vi "Read FD.vi"(8 "error in":errorcluster, 11 "TPCANHandle in":T2=81 items=["PCAN_NONEBUS"=0, "PCAN_USBBUS1"=81, "PCAN_USBBUS2"=82, "PCAN_USBBUS3"=83, "PCAN_USBBUS4"=84, "PCAN_USBBUS5"=85, "PCAN_USBBUS6"=86, "PCAN_USBBUS7"=87, "PCAN_USBBUS8"=88, "PCAN_USBBUS9"=1289, "PCAN_USBBUS10"=1290, "PCAN_USBBUS11"=1291, "PCAN_USBBUS12"=1292, "PCAN_USBBUS13"=1293, "PCAN_USBBUS14"=1294, "PCAN_USBBUS15"=1295, "PCAN_USBBUS16"=1296]) -> (0 "error out":errorcluster, 1 "Time Stamp":timestamp format="%<%x %.3X>T", 2 "PCAN Message FD":T3={"ID"=0, "MSGTYPE"={"Type"=4, "Extended"=FALSE, "ESI"=FALSE, "Echo"=FALSE}, "LEN"=enum."0", "Data"=[]} {"Data" format="%.0x"; "MSGTYPE"."Type" items=["FD"=4, "FD+BRS"=12, "ERRFRAME"=64, "STATUS"=128]}, 3 "TPCANHandle out":T2=81 items=["PCAN_NONEBUS"=0, "PCAN_USBBUS1"=81, "PCAN_USBBUS2"=82, "PCAN_USBBUS3"=83, "PCAN_USBBUS4"=84, "PCAN_USBBUS5"=85, "PCAN_USBBUS6"=86, "PCAN_USBBUS7"=87, "PCAN_USBBUS8"=88, "PCAN_USBBUS9"=1289, "PCAN_USBBUS10"=1290, "PCAN_USBBUS11"=1291, "PCAN_USBBUS12"=1292, "PCAN_USBBUS13"=1293, "PCAN_USBBUS14"=1294, "PCAN_USBBUS15"=1295, "PCAN_USBBUS16"=1296], 4 "Receive Queue empty":bool, 5 "TPCANStatus":T1 items=["PCAN_ERROR_OK"=0, "PCAN_ERROR_XMTFULL"=1, "PCAN_ERROR_OVERRUN"=2, "PCAN_ERROR_BUSLIGHT"=4, "PCAN_ERROR_BUSHEAVY"=8, "PCAN_ERROR_BUSPASSIVE"=262144, "PCAN_ERROR_BUSOFF"=16, "PCAN_ERROR_QRCVEMPTY"=32, "PCAN_ERROR_QOVERRUN"=64, "PCAN_ERROR_QXMTFULL"=128, "PCAN_ERROR_REGTEST"=256, "PCAN_ERROR_NODRIVER"=512, "PCAN_ERROR_HWINUSE"=1024, "PCAN_ERROR_NETINUSE"=2048, "PCAN_ERROR_ILLHW"=5120, "PCAN_ERROR_ILLNET"=6144, "PCAN_ERROR_ILLCLIENT"=7168, "PCAN_ERROR_RESOURCE"=8192, "PCAN_ERROR_ILLPARAMTYPE"=16384, "PCAN_ERROR_ILLPARAMVAL"=32768, "PCAN_ERROR_UNKNOWN"=65536, "PCAN_ERROR_ILLDATA"=131072, "PCAN_ERROR_ILLMODE"=524288, "PCAN_ERROR_CAUTION"=33554432, "PCAN_ERROR_INITIALIZE"=67108864, "PCAN_ERROR_ILLOPERATION"=134217728])   [LabVIEW 2020, in "PCANBasic.lvlib"]
doc: "Reads a CAN message from the receive queue of a FD capable PCAN Channel.\n\nTimestamps on Linux are the number of milliseconds that have elapsed since the epoch: the epoch is the point in time of 00:00 UTC, 1 January 1970.\n\nThe Read method returns received messages or status messages from the receive queue. It is important to call Read repeatedly until the queue is empty. In case there are no more messages in queue, the value PCAN_ERROR_QRCVEMPTY is returned. The error code PCAN_ERROR_QRCVEMPTY is also returned if the reception of messages is disabled. See Receive Status Parameter for more information. \n\nThe receive queue can contain up to 32767 messages. \n\nIf the time when the message was received is not needed, use the overloaded Read method. \n\nThere are two possibilities for reading messages from the receive queue of a Channel: \n\nTime-Triggered Reading: Consists in periodically calls to the Read method. Typically, an application starts a timer that every 50 or 100 milliseconds check for messages, calling the Read method in a loop until the value of PCAN_ERROR_QRCVEMTY or another error condition is reached. \n\nEvent-Triggered Reading: Consists in reacting to a notification sent by the PCAN driver to a registered application, when a message is received and inserted in its receive queue. See Using Events to obtain more information about reading with events. \n\nAbout bus errors / Status messages \n\nIf a bus-off error occurs, an application cannot use the channel to communicate anymore, until the CAN controller is reset. With PCAN-Basic it is not possible to reset the CAN controller through a method directly. Consider using the PCAN-Basic property PCAN_BUSOFF_AUTORESET which instructs the API to reset the CAN controller when a bus-off state is detected automatically. \n\nAnother ways to reset errors like bus-off, bus-heavy and bus-light:\n\nPerforming an uninitialize / initialize cycle: This causes a hardware reset, but only when no more clients are connected to that channel. \nUsing the parameter PCAN_HARD_RESET_STATUS: It instructs this method to explicitly perform a hardware reset regardless of whether other clients are connected to that channel. \nThe message type (see TPCANMessageType) of a CAN message indicates if the message is a 11-bit, 29-bit, RTR, Error, or Status message. This value should be checked every time a message has been read successfully. \n\nIf the bit PCAN_MESSAGE_ERRFRAME is set in the TPCANMsg.MSGTYPE field, the message is an Error frame (see Error Frames). \n\nIf the bit PCAN_MESSAGE_STATUS is set in the TPCANMsg.MSGTYPE field, the message is a Status message. The ID and LEN fields do not contain valid data. The first 4 data bytes of the message contain the Error Code. The MSB of the Error Code is in data byte 0, the LSB is in data byte 3."
uses:
  PCANBasic.lvlib
  Data Length Code FD.ctl
  TPCANStatus.ctl
  kernel32.dll
  peak/PCANBasic64.dll
  TPCANHandle.ctl
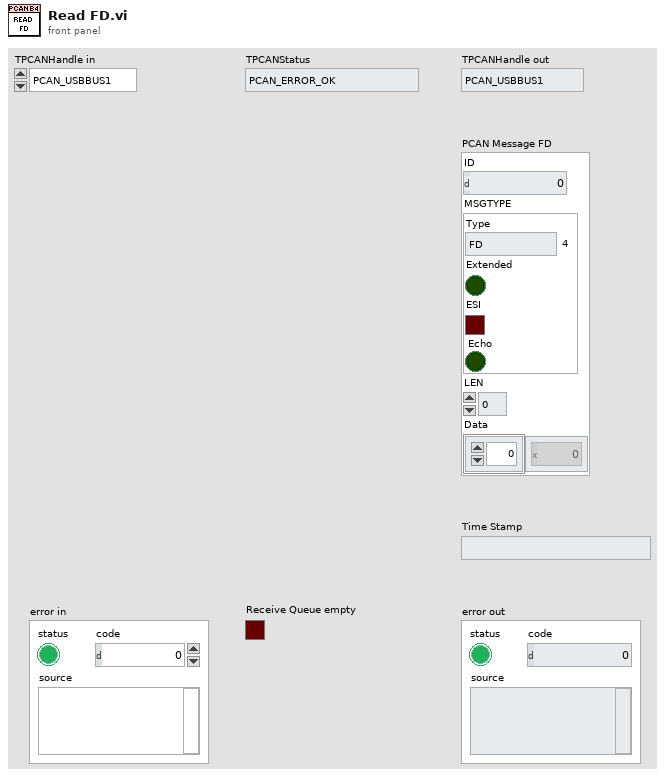
[diagram p1: front panel]
types:
  T1 = typedef "PCANBasic.lvlib/TPCANStatus.ctl" = u32
  T2 = typedef "PCANBasic.lvlib/TPCANHandle.ctl" = u16
  T3 = cluster{"ID":u32, "MSGTYPE":cluster{"Type":u8, "Extended":bool, "ESI":bool, "Echo":bool}, "LEN":enum8{"0", "1", "2", "3", "4", "5", "6", "7", "8", "12", "16", "20", "24", "32", "48", "64"}, "Data":u8[]}
  T4 = typedef "PCANBasic.lvlib/Data Length Code FD.ctl" = enum8{"0", "1", "2", "3", "4", "5", "6", "7", "8", "12", "16", "20", "24", "32", "48", "64"}
  T5 = cluster{"ID":u32, "MSGTYPE":cluster{"Type":u8, "Extended":bool, "ESI":bool, "Echo":bool}, "LEN":T4, "Data":u8[]}
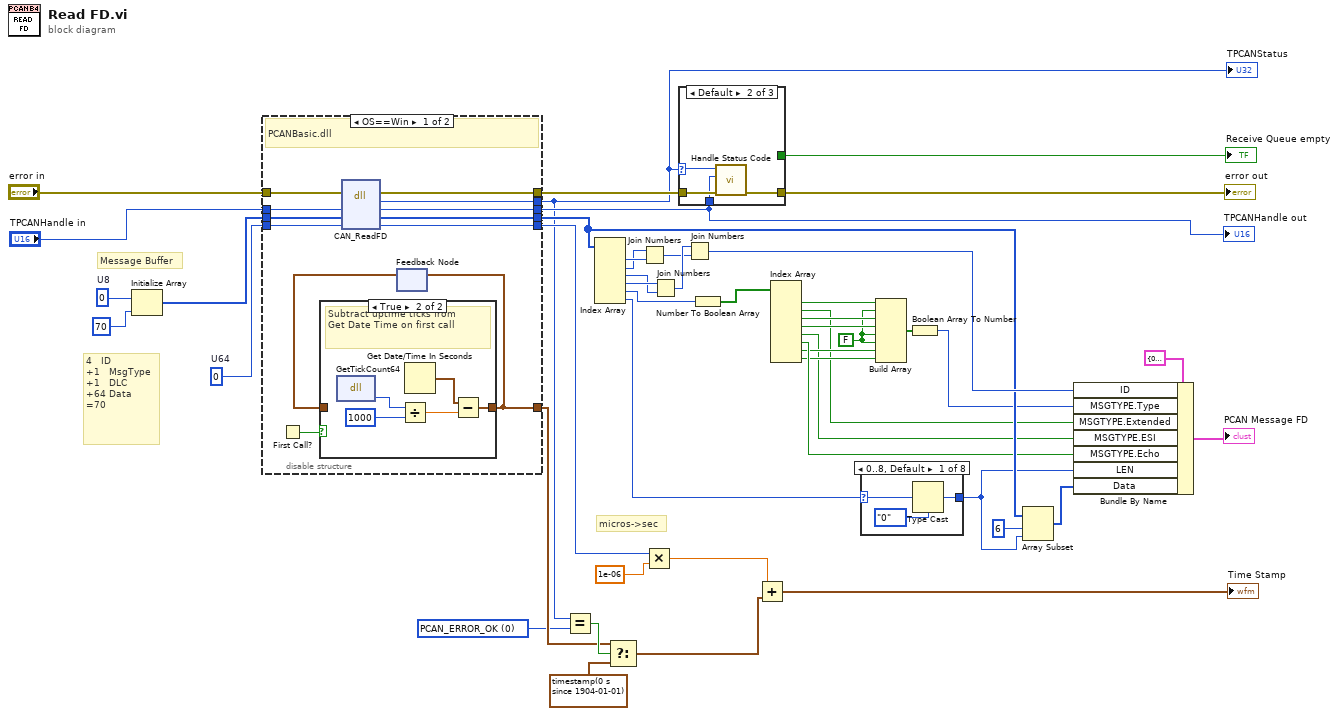
[diagram p0: block diagram]
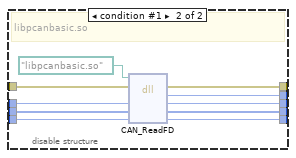
[diagram p3: hidden frame]
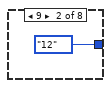
[diagram p4: hidden frame]
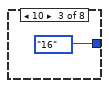
[diagram p5: hidden frame]
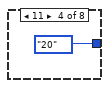
[diagram p6: hidden frame]
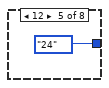
[diagram p7: hidden frame]
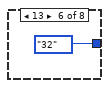
[diagram p8: hidden frame]
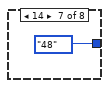
[diagram p9: hidden frame]
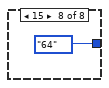
[diagram p10: hidden frame]
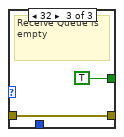
[diagram p12: hidden frame]
diagram:
  w1 = T1 0 items=["PCAN_ERROR_OK"=0, "PCAN_ERROR_XMTFULL"=1, "PCAN_ERROR_OVERRUN"=2, "PCAN_ERROR_BUSLIGHT"=4, "PCAN_ERROR_BUSHEAVY"=8, "PCAN_ERROR_BUSPASSIVE"=262144, "PCAN_ERROR_BUSOFF"=16, "PCAN_ERROR_QRCVEMPTY"=32, "PCAN_ERROR_QOVERRUN"=64, "PCAN_ERROR_QXMTFULL"=128, "PCAN_ERROR_REGTEST"=256, "PCAN_ERROR_NODRIVER"=512, "PCAN_ERROR_HWINUSE"=1024, "PCAN_ERROR_NETINUSE"=2048, "PCAN_ERROR_ILLHW"=5120, "PCAN_ERROR_ILLNET"=6144, "PCAN_ERROR_ILLCLIENT"=7168, "PCAN_ERROR_RESOURCE"=8192, "PCAN_ERROR_ILLPARAMTYPE"=16384, "PCAN_ERROR_ILLPARAMVAL"=32768, "PCAN_ERROR_UNKNOWN"=65536, "PCAN_ERROR_ILLDATA"=131072, "PCAN_ERROR_ILLMODE"=524288, "PCAN_ERROR_CAUTION"=33554432, "PCAN_ERROR_INITIALIZE"=67108864, "PCAN_ERROR_ILLOPERATION"=134217728] ("TPCANStatus 2")
  w12 = FALSE
  w38 = u8 0  # U8
  w41 = u64 0  # U64
  # "4   ID\n+1   MsgType\n+1   DLC\n+64 Data\n=70"
  # "Message Buffer"
  # "micros->sec"
  n1 = Initialize Array(w38, 70 ("dimension size")) -> (w28:u8[])
  n2 = disable-structure shown="OS==Win" {
    disable-tunnel: "error in" -> [w59 w75]
    disable-tunnel: [w58 w74] -> w46
    disable-tunnel: "TPCANHandle in" -> [w57 w73]
    disable-tunnel: [w56 w72] -> w2
    disable-tunnel: [w55 w71] -> w42
    disable-tunnel: w41 -> [w54 w70]
    disable-tunnel: [w53 w69] -> w39
    disable-tunnel: w28 -> [w52 w68]
    disable-tunnel: [w51 w67] -> w26
    disable-tunnel: [w48 _] -> w4
    frame condition #0 (active) {
      # "PCANBasic.dll"
      n3 = First Call?() -> (First Call?: T/F=w50:bool)
      n4 = dll-call lib="D:/git/PCAN-Basic-LabVIEW/source/peak/PCANBasic*.dll" fn="CAN_ReadFD"(error in=w59, "Channel"=w57, "MessageBuffer"=w52, "TimestampBuffer"=w54) -> (error out=w58:errorcluster, "TPCANStatus"=w56:u32, "Channel"=w55:u16, "MessageBuffer"=w51:u8[], "TimestampBuffer"=w53:u64)  [unwired: 2 in, 1 out]
      n5 = feedback #1() -> (w49:timestamp)  [unwired: 1 in]
      n6 = case shown="True" w50 {
        tunnel: [w60 w61] -> w48
        tunnel: w49 -> [w60 _]
        frame False {
          # "forward value of first call"
        }
        frame True {
          # "Subtract uptime ticks from\nGet Date Time on first call"
          n7 = dll-call lib="kernel32.dll" fn="GetTickCount64"() -> ("return type"=w65:u64)  [unwired: 3 in, 2 out]
          n8 = Divide(x=w65, y=u64 1000) -> (x/y=w62:dbl)
          n9 = Get Date/Time In Seconds() -> (seconds since 1Jan1904=w63:timestamp)
          n10 = Subtract(x=w63, y=w62) -> (x-y=w61:timestamp)
        }
      }
      n11 = feedback-in #1(w48) -> ()
    }
    frame condition #1 {
      # "libpcanbasic.so"
      n12 = dll-call lib="?" fn="CAN_ReadFD"(path in=path "libpcanbasic.so", error in=w75, "Channel"=w73, "MessageBuffer"=w68, "TimestampBuffer"=w70) -> (error out=w74:errorcluster, "TPCANStatus"=w72:u32, "Channel"=w71:u16, "MessageBuffer"=w67:u8[], "TimestampBuffer"=w69:u64)  [unwired: 1 in, 1 out]
    }
  }
  "TPCANHandle out" <- w42
  "TPCANStatus" <- w2
  n13 = Equal?(x=w2, y=w1) -> (x = y?=w6:bool)
  n14 = Index Array(array=w26) -> (element #1=w34:u8, element #2=w33:u8, element #3=w31:u8, element #4=w32:u8, element #5=w11:u8, element #6=w29:u8)  [unwired: 6 in]
  n15 = Select(t=w4, s=w6, f=timestamp(0 s since 1904-01-01)) -> (s? t:f=w3:timestamp)
  n16 = Join Numbers(hi=w33, lo=w34) -> ((hi.lo)=w35:u16)
  n17 = Multiply(x=w39, y=1e-06) -> (x*y=w23:dbl)
  n18 = Join Numbers(hi=w32, lo=w31) -> ((hi.lo)=w36:u16)
  n19 = case shown="Default" w2 {
    selector: w2 -> [_ w78 _]
    tunnel: w46 -> [w76 w80 w82]
    tunnel: [w76 w79 w82] -> w45
    tunnel: [_ _ TRUE] -> w44
    tunnel: w42 -> [_ w77 _]
    frame 0 {
    }
    frame Default {
      n20 = call "Handle Status Code.vi"("error in"=w80, "TPCANHandle"=w77, "TPCANStatus"=w78) -> ("error out"=w79:errorcluster)  [unwired: 8 in]
    }
    frame 32 {
      # "Receive Queue is empty"
    }
  }
  "error out" <- w45
  "Receive Queue empty" <- w44
  n21 = Join Numbers(hi=w36, lo=w35) -> ((hi.lo)=w30:u32)
  n22 = Number To Boolean Array(number=w11) -> (Boolean array=w21:bool[])
  n23 = Add(x=w23, y=w3) -> (x+y=→"Time Stamp":timestamp)
  n24 = Index Array(array=w21) -> (element #1=w17:bool, element #2=w13:bool, element #3=w16:bool, element #4=w15:bool, element #5=w14:bool, element #6=w20:bool, element #7=w18:bool, element #8=w19:bool)  [unwired: 8 in]
  n25 = case "DLC" shown="0..8, Default" w29 {
    selector: w29 -> [w85 _ _ _ _ _ _ _]
    tunnel: [w84 Data_Length_Code_FD."12" ("LEN") Data_Length_Code_FD."16" ("LEN") Data_Length_Code_FD."20" ("LEN") Data_Length_Code_FD."24" ("LEN") Data_Length_Code_FD."32" ("LEN") Data_Length_Code_FD."48" ("LEN") Data_Length_Code_FD."64" ("LEN")] -> w25
    frame 0..8, Default {
      n26 = Type Cast(type=Data_Length_Code_FD."0" ("LEN"), x=w85) -> (*(type *) &x=w84:T4)
    }
    frame 9 {
    }
    frame 10 {
    }
    frame 11 {
    }
    frame 12 {
    }
    frame 13 {
    }
    frame 14 {
    }
    frame 15 {
    }
  }
  n27 = Build Array(w17, w12, w16, w15, w12, w12, w18, w19) -> (w10:bool[])
  n28 = Boolean Array To Number(Boolean array=w10) -> (number=w9:u32)
  n29 = Array Subset(array=w26, index=6, length=w25) -> (w24:u8[])
  n30 = Bundle By Name(cluster=T5 {"ID"=0, "MSGTYPE"={"Type"=4, "Extended"=FALSE, "ESI"=FALSE, "Echo"=FALSE}, "LEN"=enum."0", "Data"=[]} ("PCAN Message FD"), "ID"=w30, "MSGTYPE.Type"=w9, "MSGTYPE.Extended"=w13, "MSGTYPE.ESI"=w14, "MSGTYPE.Echo"=w20, "LEN"=w25, "Data"=w24) -> (→"PCAN Message FD":T5)
